vi "Update Asset Metadata.vi"(4 "Value":string="bar", 6 "Property":string="foo", 8 "error in (no error)":errorcluster, 10 "Serial Number":string="1234", 11 "Part Number":string="B0CG1KL3RC") -> (0 "error out":errorcluster, 3 "asset id":string="2d7e2a0f-e140-47e2-ae68-ae9bd23d949b")   [LabVIEW 2024]
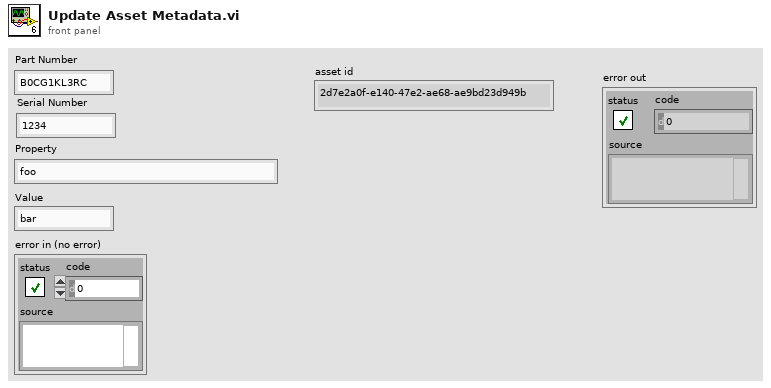
[diagram p1: front panel]
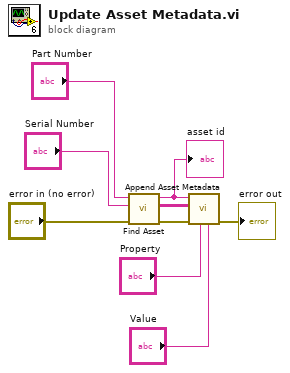
[diagram p0: block diagram]
diagram:
  n1 = call "Find Asset.vi"("error in (no error)"="error in (no error)", "Serial Number"="Serial Number", "Part Number"="Part Number") -> ("error out"=w6:errorcluster, "Properties"=w3:string[][], "Asset ID"=w4:string)  [unwired: 6 in]
  "asset id" <- w4
  n2 = call "Append Asset Metadata.vi"("Value"="Value", "Property"="Property", "error in (no error)"=w6, "Properties"=w3, "Asset ID"=w4) -> ("error out"=→"error out":errorcluster)  [unwired: 6 in]
